vi "Init.vi"(8 "error in (no error)":errorcluster, 11 "Videoscan in":refnum<class "Videoscan.lvclass">) -> (0 "error out":errorcluster, 3 "Videoscan out":refnum<class "Videoscan.lvclass">)   [LabVIEW 2014, in "Videoscan.lvclass"]
uses:
  Videoscan.lvclass
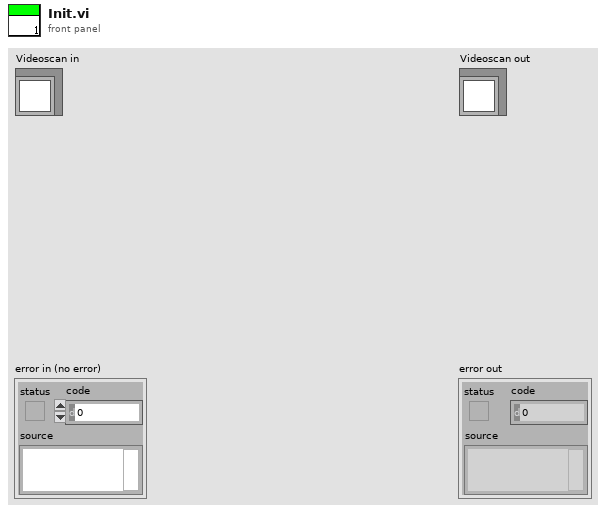
[diagram p1: front panel]
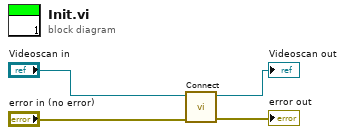
[diagram p0: block diagram]
diagram:
  n1 = call-dynamic "Connect.vi"("error in (no error)"="error in (no error)", "Videoscan in"="Videoscan in") -> ("error out"=→"error out":errorcluster, "Videoscan out"=→"Videoscan out":refnum<class "Videoscan.lvclass">)  [unwired: 8 in]
